vi "Timing Engine Unit Test Main.vi"   [LabVIEW 2016, in "Assert API Components.lvlib" / "Assert Display.lvlib" / "Timing Engine Tester.lvlib"]
uses:
  Timing Engine Tester.lvlib
  Timing Engine Tester/Timing Engine Tester.lvclass
  C:/Program Files (x86)/National Instruments/LabVIEW 2016/vi.lib/ActorFramework/Actor/Actor.lvclass
  <vilib>/ActorFramework/Actor/Actor.lvclass
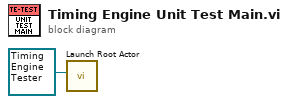
[diagram p0: block diagram]
diagram:
  n1 = call <vilib>:"Launch Root Actor.vi"("Actor"=refnum<class "Timing Engine Tester.lvclass"> refnum ("Assert API Components.lvlib:Assert Display.lvlib:Timing Engine Tester.lvlib:Timing Engine Tester.lvclass")) -> ()  [unwired: 9 in, 2 out]
